vi "Auton Parse Scripts.vi"(11 "Array":dbl[][](array[numeric])) -> ()   [LabVIEW 2016]
uses:
  Common Code/Auton Command Cluster.ctl
  Robot Global Data.vi
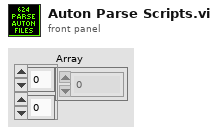
[diagram p1: front panel]
types:
  T1 = typedef "Auton Command Cluster.ctl" = cluster{"commandID":dbl, "maxTime":dbl, "distanceTarget":dbl, "headingTarget":dbl, "translationTarget":dbl, "ySpeed":dbl, "xSpeed":dbl, "zSpeed":dbl, "async":dbl, "RPM":dbl, "Hood?":dbl, "Hopper?":dbl, "rollerPower":dbl, "fillHopper?":dbl, "zeroGyro":dbl}
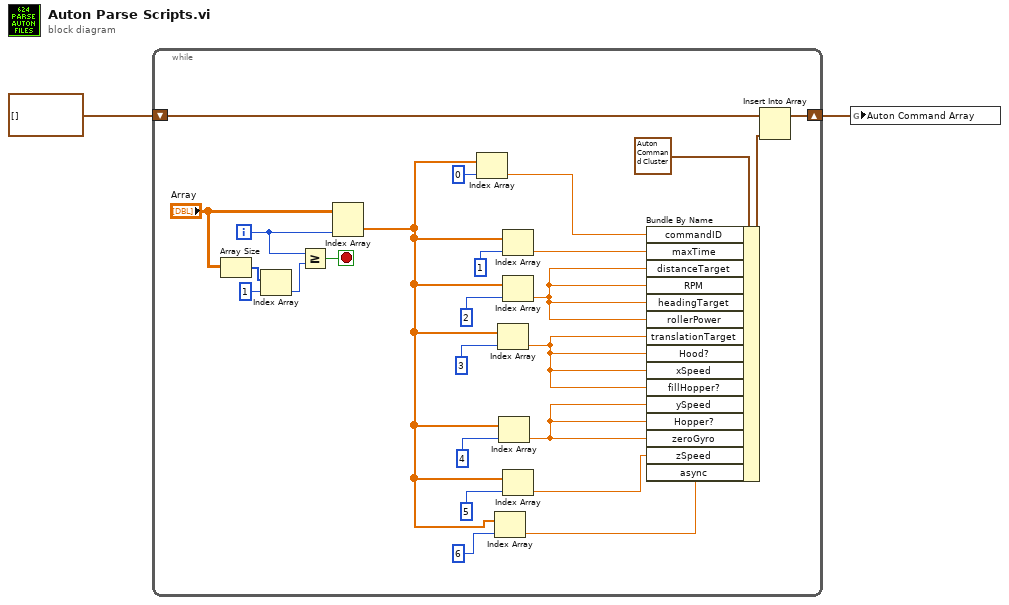
[diagram p0: block diagram]
diagram:
  n1 = while {
    shift-right: [w27] -> w1
    shift-left: T1[] [] ("Auton Command Array") -> [w26]
    i -> [w21]
    stop <- w20 stop-if-true
    n2 = Array Size(array="Array") -> (size(s)=w24:i32[])
    n3 = Index Array(array=w24, index=1) -> (element=w22:i32)
    n4 = Greater Or Equal?(x=w21, y=w22) -> (x >= y?=w20:bool)
    n5 = Index Array(array="Array", index (col)=w21) -> (element=w12:dbl[])  [unwired: 1 in]
    n6 = Index Array(array=w12, index=0) -> (element=w9:dbl)
    n7 = Index Array(array=w12, index=6) -> (element=w3:dbl)
    n8 = Index Array(array=w12, index=3) -> (element=w6:dbl)
    n9 = Index Array(array=w12, index=4) -> (element=w5:dbl)
    n10 = Index Array(array=w12, index=1) -> (element=w8:dbl)
    n11 = Index Array(array=w12, index=2) -> (element=w7:dbl)
    n12 = Index Array(array=w12, index=5) -> (element=w4:dbl)
    n13 = Bundle By Name(cluster=T1 {"commandID"=0.0, "maxTime"=0.0, "distanceTarget"=0.0, "headingTarget"=0.0, "translationTarget"=0.0, "ySpeed"=0.0, "xSpeed"=0.0, "zSpeed"=0.0, "async"=0.0, "RPM"=0.0, "Hood?"=0.0, "Hopper?"=0.0, "rollerPower"=0.0, "fillHopper?"=0.0, "zeroGyro"=0.0} ("Cluster"), "commandID"=w9, "maxTime"=w8, "distanceTarget"=w7, "RPM"=w7, "headingTarget"=w7, "rollerPower"=w7, "translationTarget"=w6, "Hood?"=w6, "xSpeed"=w6, "fillHopper?"=w6, "ySpeed"=w5, "Hopper?"=w5, "zeroGyro"=w5, "zSpeed"=w4, "async"=w3) -> (w10:T1)
    n14 = Insert Into Array(array=w26, new element=w10) -> (w27:T1[])  [unwired: 1 in]
  }
  n15 = global write "Robot Global Data.vi" "Auton Command Array"(w1) -> ()
